vi "InitiateNotifiers.vi"() -> (1 "Notifiers":T1)   [LabVIEW 2012]
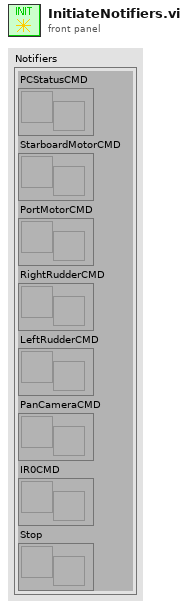
[diagram p1: front panel]
types:
  T1 = cluster{"PCStatusCMD":refnum<notifier>, "StarboardMotorCMD":refnum<notifier>, "PortMotorCMD":refnum<notifier>, "RightRudderCMD":refnum<notifier>, "LeftRudderCMD":refnum<notifier>, "PanCameraCMD":refnum<notifier>, "IR0CMD":refnum<notifier>, "Stop":refnum<notifier>}
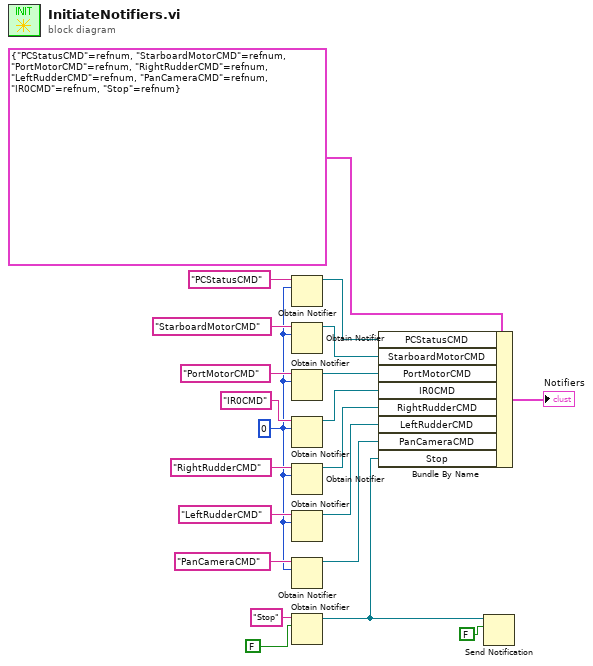
[diagram p0: block diagram]
diagram:
  w14 = 0 ("Port\nMotor")
  n1 = Obtain Notifier(name (unnamed)="PCStatusCMD", notification data type=w14) -> (notifier out=w12:refnum<notifier>)  [unwired: 2 in, 2 out]
  n2 = Obtain Notifier(name (unnamed)="StarboardMotorCMD", notification data type=w14) -> (notifier out=w11:refnum<notifier>)  [unwired: 2 in, 2 out]
  n3 = Obtain Notifier(name (unnamed)="PortMotorCMD", notification data type=w14) -> (notifier out=w10:refnum<notifier>)  [unwired: 2 in, 2 out]
  n4 = Obtain Notifier(name (unnamed)="IR0CMD", notification data type=w14) -> (notifier out=w9:refnum<notifier>)  [unwired: 2 in, 2 out]
  n5 = Obtain Notifier(name (unnamed)="RightRudderCMD", notification data type=w14) -> (notifier out=w8:refnum<notifier>)  [unwired: 2 in, 2 out]
  n6 = Obtain Notifier(name (unnamed)="LeftRudderCMD", notification data type=w14) -> (notifier out=w7:refnum<notifier>)  [unwired: 2 in, 2 out]
  n7 = Obtain Notifier(name (unnamed)="PanCameraCMD", notification data type=w14) -> (notifier out=w6:refnum<notifier>)  [unwired: 2 in, 2 out]
  n8 = Obtain Notifier(name (unnamed)="Stop", notification data type=FALSE ("Boolean")) -> (notifier out=w2:refnum<notifier>)  [unwired: 2 in, 2 out]
  n9 = Bundle By Name(cluster=T1 {"PCStatusCMD"=refnum, "StarboardMotorCMD"=refnum, "PortMotorCMD"=refnum, "RightRudderCMD"=refnum, "LeftRudderCMD"=refnum, "PanCameraCMD"=refnum, "IR0CMD"=refnum, "Stop"=refnum} ("input cluster"), "PCStatusCMD"=w12, "StarboardMotorCMD"=w11, "PortMotorCMD"=w10, "IR0CMD"=w9, "RightRudderCMD"=w8, "LeftRudderCMD"=w7, "PanCameraCMD"=w6, "Stop"=w2) -> (→"Notifiers":T1)
  n10 = Send Notification(notification=FALSE, notifier=w2) -> ()  [unwired: 1 in, 2 out]
